vi "Reset.vi"(6 "Reset Mode":T1, 8 "error in (no error)":errorcluster, 9 "Files to Reset":path[](array[path]), 10 "Target":string="HEAD" caption="Target (HEAD)", 11 "Git Implementation in":refnum<class "Git Implementation.lvclass">) -> (0 "error out":errorcluster, 2 "Status Message":string, 3 "Git Implementation out":refnum<class "Git Implementation.lvclass">)   [LabVIEW 2017, in "Git-LabVIEW.lvlib" / "Git Implementation.lvclass"]
doc: "Reset the state of the repository based on the Reset Mode and the current state.\nHard will modify the local directory to match the Target.\nSoft will not modify the local directory, but will update HEAD.\nMixed will move the HEAD to the Target, and update the index, but will not change the local directory contents.\n\nAlternatively files can be specified to be reset - in this case, the file copies will be copied from Target to the index (what would be commited if a 'Git Commit' immediately followed)."
uses:
  Git Implementation.lvclass
  Reset Mode.ctl
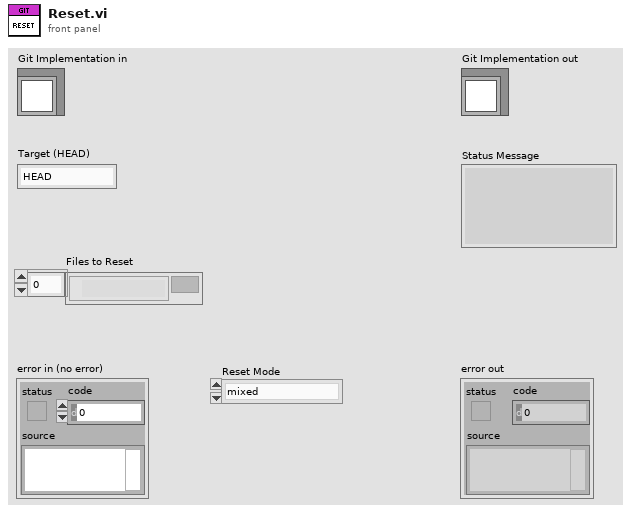
[diagram p1: front panel]
types:
  T1 = typedef "Git-LabVIEW.lvlib/Git Implementation.lvclass/Reset Mode.ctl" = enum16{"mixed", "soft", "hard", "merge", "keep"}
  T2 = typedef "Git-LabVIEW.lvlib/Git Implementation.lvclass/CMD Return.ctl" = cluster{"StdOut":string, "StdErr":string, "Return Code":i32}
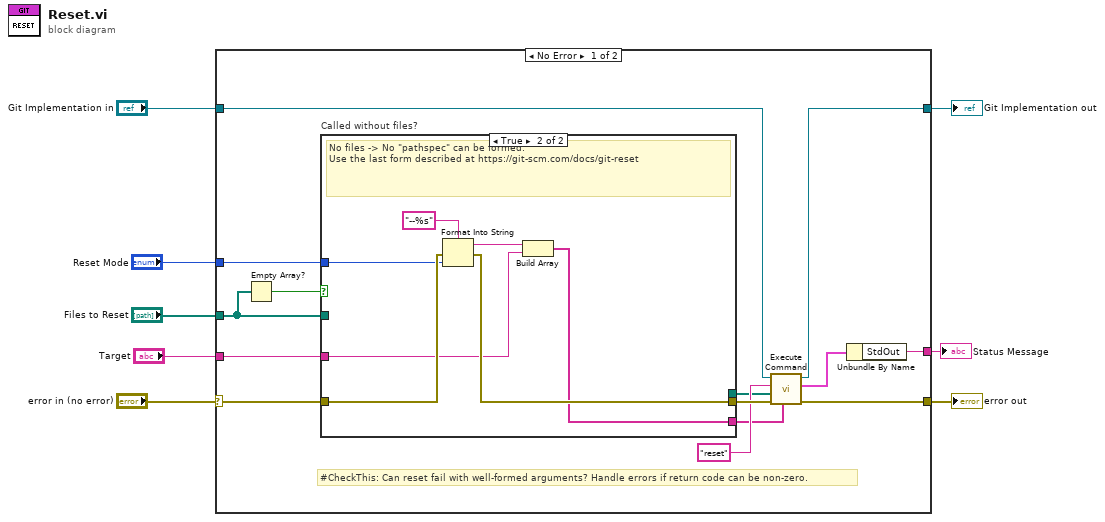
[diagram p0: block diagram]
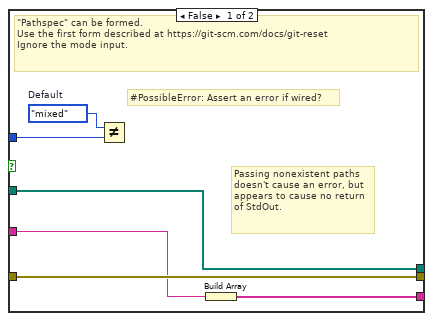
[diagram p2: hidden frame]
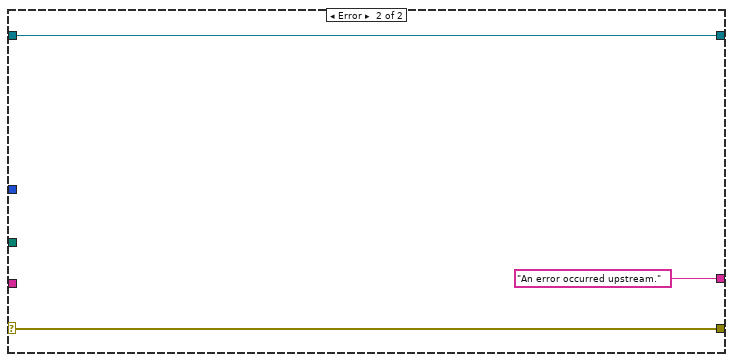
[diagram p3: hidden frame]
diagram:
  n1 = case shown="No Error" "error in (no error)" {
    selector: "error in (no error)" -> [w18 w38]
    tunnel: [w17 w38] -> w7
    tunnel: [w14 w37] -> w5
    tunnel: "Git Implementation in" -> [w15 w37]
    tunnel: "Files to Reset" -> [w21 _]
    tunnel: "Target" -> [w20 _]
    tunnel: "Reset Mode" -> [w19 _]
    tunnel: [w9 "An error occurred upstream." ("StdOut")] -> w1
    frame No Error {
      # "#CheckThis: Can reset fail with well-formed arguments? Handle errors if return code can be non-zero."
      n2 = Empty Array?(array=w21) -> (empty?=w22:bool)
      n3 = case "Called without files?" shown="True" w22 {
        tunnel: w21 -> [w25 _]
        tunnel: w20 -> [w24 w29]
        tunnel: w19 -> [w28 w33]
        tunnel: w18 -> [w26 w35]
        tunnel: [w26 w34] -> w16
        tunnel: [w25 _] -> w12
        tunnel: [w23 w30] -> w11
        frame False {
          w27 = Reset_Mode."mixed"  # Default
          # "Passing nonexistent paths doesn't cause an error, but appears to cause no return of StdOut."
          # "#PossibleError: Assert an error if wired?"
          # "\"Pathspec\" can be formed. \nUse the first form described at https://git-scm.com/docs/git-reset\nIgnore the mode input."
          n4 = Not Equal?(x=w27, y=w28) -> ()  [unwired: 1 out]
          n5 = Build Array(w24) -> (w23:string[])
        }
        frame True {
          # "No files -> No \"pathspec\" can be formed.\nUse the last form described at https://git-scm.com/docs/git-reset"
          n6 = Format Into String(format string="--%s", error in=w35, w33) -> (resulting string=w31:string, error out=w34:errorcluster)  [unwired: 1 in]
          n7 = Build Array(w31, w29) -> (w30:string[])
        }
      }
      n8 = call "Execute Command.vi"("Arguments"=w11, "error in (no error)"=w16, "File Paths"=w12, "Command"="reset", "Git Implementation in"=w15) -> ("error out"=w17:errorcluster, "CMD Return"=w10:T2, "Git Implementation out"=w14:refnum<class "Git Implementation.lvclass">)  [unwired: 4 in]
      n9 = Unbundle By Name(w10) -> ("StdOut"=w9:string)
    }
    frame Error {
    }
  }
  "error out" <- w7
  "Git Implementation out" <- w5
  "Status Message" <- w1
